vi "lv9_daqusb6251.vi"() -> ()   [LabVIEW 2009]
panel:
  in  "Measures numbers":u32=3
  in  "Filename":path=path "test.lvm"
  in  "Enable save data":bool=TRUE caption="Enable"
  out "x-y":u32
  in  "number of samples":i32=1
  in  "Loop Time [ms]":u32=50
  out "Dinamometro":string
  in  "VISA resource name":refnum<visa-resource-name>="COM4"
  out "Iteration":i32
  out "Waveform Chart 2":dynamicdata(graph)=[{"t0"=timestamp(3730382840.471822 s since 1904-01-01), "dt"=1.0, "Y"=[-0.00023800805463109788]}]
  in  "Device name":tag="Dev1"
  in  "Number of samples \nto read":i32=-1
  out "Waveform Chart":dynamicdata(graph)=[{"t0"=timestamp(3730382840.471822 s since 1904-01-01), "dt"=1.0, "Y"=[-0.23734714614383248]}]
  in  "Stop":bool
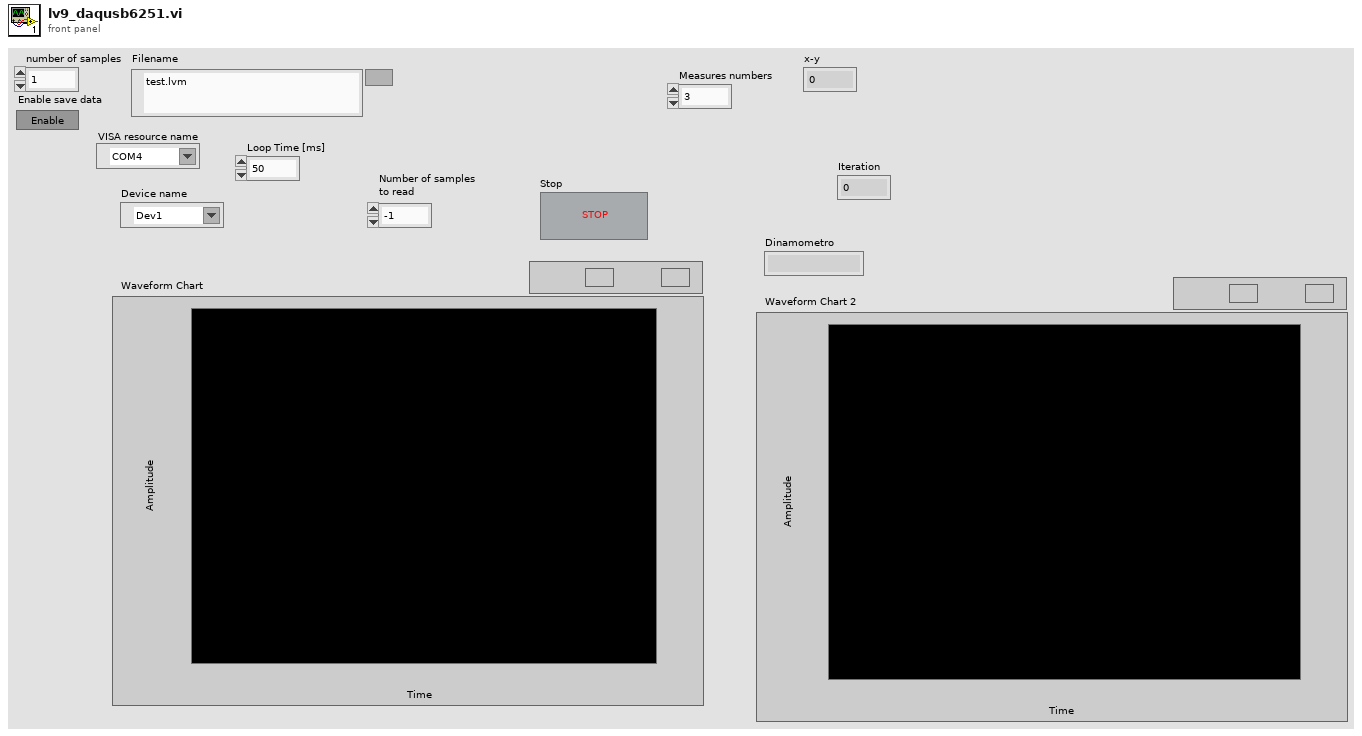
[diagram p1: front panel]
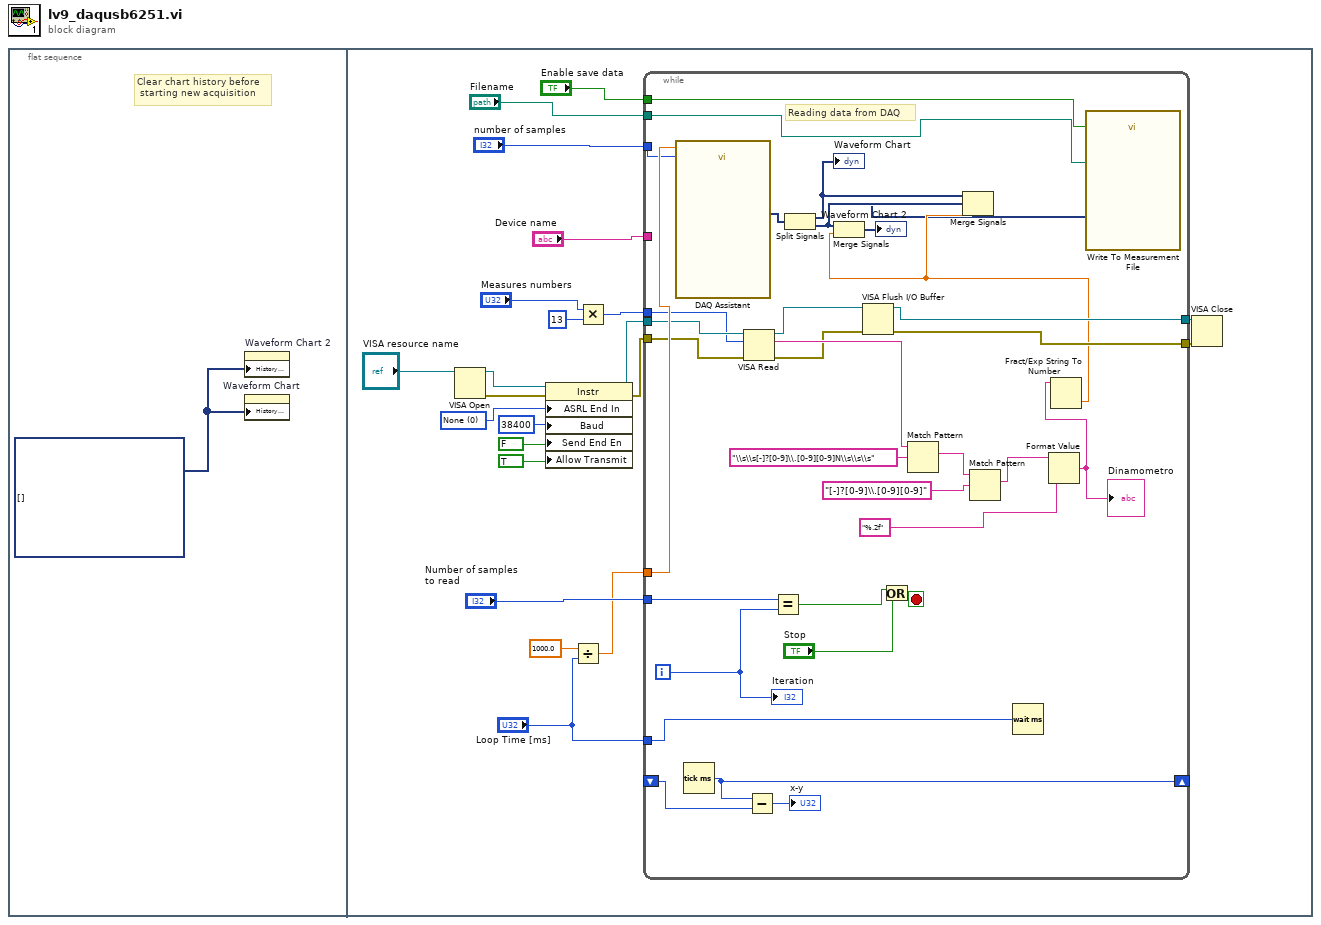
[diagram p0: block diagram]
diagram:
  n1 = flat-sequence {
    frame #0 {
      w1 = dynamicdata[] [] ("History Data")
      # "Clear chart history before\n starting new acquisition"
      n2 = property on="Waveform Chart 2" class="WFChart (strict)"("History Data"=w1) -> ()  [unwired: 2 in, 2 out]
      n3 = property on="Waveform Chart" class="WFChart (strict)"("History Data"=w1) -> ()  [unwired: 2 in, 2 out]
    }
    frame #1 {
      w15 = u16 0 items=["None", "Last Bit", "TermChar"] ("Serial Settings:End Mode for Reads")
      n4 = VISA Open(VISA resource name="VISA resource name") -> (VISA resource name=w17:refnum<visa-resource-name>, error out=w18:errorcluster)  [unwired: 4 in]
      n5 = property class="Instr"(reference=w17, error in=w18, "ASRL End In"=w15, "Baud"=u32 38400 ("Serial Settings:Baud Rate"), "Send End En"=FALSE, "Allow Transmit"=TRUE) -> (reference out=w20:refnum<visa-resource-name>, error out=w19:errorcluster)
      n6 = Divide(x=1000.0, y="Loop Time [ms]") -> (x/y=w11:dbl)
      n7 = Multiply(x="Measures numbers", y=u32 13) -> (x*y=w3:u32)
      n8 = while {
        tunnel: "Device name" -> [_]
        tunnel: "Number of samples \nto read" -> [w52]
        tunnel: w20 -> [w39]
        tunnel: w19 -> [w38]
        tunnel: "Loop Time [ms]" -> [w47]
        tunnel: w11 -> [w46]
        tunnel: [w42] -> w10
        tunnel: [w41] -> w9
        tunnel: "number of samples" -> [w37]
        shift-right: [w35] -> _
        shift-left: _ -> [w34]
        tunnel: "Enable save data" -> [w26]
        tunnel: "Filename" -> [w25]
        tunnel: w3 -> [w24]
        i -> [w54]
        stop <- w55 stop-if-true
        # "Reading data from DAQ"
        n9 = call "DAQ Assistant"("rate"=w46, "number of samples"=w37) -> ("data"=w49:dynamicdata)  [unwired: 14 in, 3 out]
        n10 = Tick Count (ms)() -> (millisecond timer value=w35:u32)
        n11 = VISA Read(VISA resource name=w39, byte count=w24, error in (no error)=w38) -> (VISA resource name out=w43:refnum<visa-resource-name>, read buffer=w45:string, error out=w40:errorcluster)  [unwired: 1 out]
        n12 = Subtract(x=w35, y=w34) -> (x-y=→"x-y":u32)
        n13 = Equal?(x=w52, y=w54) -> (x = y?=w53:bool)
        n14 = Split Signals(w49) -> (w30:dynamicdata, w29:dynamicdata)  [unwired: 2 in]
        "Waveform Chart" <- w30
        n15 = VISA Flush I/O Buffer(VISA resource name=w43, error in (no error)=w40) -> (VISA resource name out=w42:refnum<visa-resource-name>, error out=w41:errorcluster)  [unwired: 1 in]
        n16 = Or(x=w53, y="Stop") -> (x .or. y?=w55:bool)
        n17 = Match Pattern(string=w45, regular expression="\\s\\s[-]?[0-9]\\.[0-9][0-9]N\\s\\s\\s") -> (match substring=w33:string)  [unwired: 1 in, 3 out]
        n18 = Match Pattern(string=w33, regular expression="[-]?[0-9]\\.[0-9][0-9]") -> (match substring=w31:string)  [unwired: 1 in, 3 out]
        n19 = Wait (ms)(milliseconds to wait=w47) -> ()  [unwired: 1 out]
        n20 = Format Value(string ("")=w31, format string="%.2f") -> (output string=w50:string)  [unwired: 1 in]
        "Dinamometro" <- w50
        n21 = Fract/Exp String To Number(string=w50) -> (number=w28:dbl)  [unwired: 3 in, 1 out]
        n22 = Merge Signals(w29, w28) -> (→"Waveform Chart 2":dynamicdata)
        n23 = Merge Signals(w30, w29, w28) -> (w27:dynamicdata)
        n24 = call "Write To Measurement File"("Signals"=w27, "Enable"=w26, "Filename"=w25) -> ()  [unwired: 14 in, 3 out]
        "Iteration" <- w54
      }
      n25 = VISA Close(VISA resource name=w10, error in (no error)=w9) -> ()  [unwired: 1 out]
    }
  }
